vi "PH_BL-Master.ProcEvents.vi"(0 "i ref in":refnum<vi>, 5 "error in (no error)":errorcluster) -> (14 "i ref out":refnum<vi>, 19 "error out":errorcluster)   [LabVIEW 2014, in "PH_BL-Master.lvlib"]
doc: "This method is used to define the events the object will listen to. Add your own events here."
uses:
  PH_BL-Master.lvlib
  CSCore/BaseProcess/BaseProcess.event definition.ctl
  CSCore/CAEObj/CAEObj.event definition.ctl
  CSCore/BaseProcess/BaseProcess.descriptor string definition.ctl
  CSCore/BaseProcess/BaseProcess.lvlib
  CSCore/CAEObj/CAEObj.lvlib
  PH_Common/PH_Common.lvlib
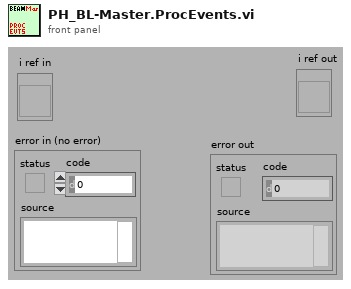
[diagram p1: front panel]
types:
  T1 = typedef "BaseProcess.lvlib/BaseProcess.event definition.ctl" = cluster{"CAEEvtDef":T2, "Data Descriptor":T3}
  T2 = typedef "CAEObj.lvlib/CAEObj.event definition.ctl" = cluster{"URL":string, "enable":bool, "ignoreResID":bool}
  T3 = typedef "BaseProcess.lvlib/BaseProcess.descriptor string definition.ctl" = string
  T4 = typedef "PH_BL-Master.lvlib/PH_BL-Master.i attribute.ctl" = cluster{"Remote controlled":bool, "Boolean Condition Service Subscriber":refnum<vi>[], "Picture Condition Service Subscriber":refnum<vi>[], "R2S":cluster{"GUI Ref":refnum<vi>, "State":bool}, "Vacua":cluster{"GUI Ref":refnum<vi>, "Limit":dbl, "Curr Value":dbl, "in range":bool}[], "O2 Inspection":cluster{"GUI Ref":refnum<vi>, "Concentration":dbl, "State":T5}[], "Boolean Status Service Subscriber":cluster{"GUI Ref":refnum<vi>, "Status":T5, "no Link?":bool, "Status Subscriber Class":T6}[], "Picture Status Service Subscriber":cluster{"GUI Ref":refnum<vi>, "Status":T5, "no Link?":bool, "Status Subscriber Class":T6}[], "6P 4Q Service Subscriber":cluster{"GUI Ref":refnum<vi>, "Selector":T7, "no Link?":bool}[], "Index of latest 6P 4Q changing Instance":i32, "Index of latest Picture Status changing Instance":i32, "Index of latest Boolean Status changing Instance":i32, "Vision ID on same Node":string, "Start Phase over?":bool, "GUI Ref Delete":refnum<vi>}
  T5 = typedef "PH_StatusHandler.lvlib/PH_StatusHandler.Status.ctl" = i16
  T6 = typedef "PH_BL-Master.lvlib/PH_BL-Master.Status Subscriber Class.ctl" = enum16{"unknown", "Switch", "BB", "6P Switch", "Switch GUI", "Switch and 6P State", "Force Sensor"}
  T7 = typedef "PH_4_Pos_Selector.lvlib/PH_4_Pos_Selector.Position Selector.ctl" = u16
  T8 = cluster{"GUI Ref":refnum<vi>, "Limit":dbl, "Curr Value":dbl, "in range":bool}[]
  T9 = cluster{"GUI Ref":refnum<vi>, "Selector":T7, "no Link?":bool}[]
  T10 = cluster{"GUI Ref":refnum<vi>, "Concentration":dbl, "State":T5}[]
  T11 = cluster{"GUI Ref":refnum<vi>, "Status":T5, "no Link?":bool, "Status Subscriber Class":T6}[]
  T12 = typedef "PH_Common.lvlib/PH_DIM.Event Declarer.ctl" = cluster{"Service Name":string, "Selector":string}
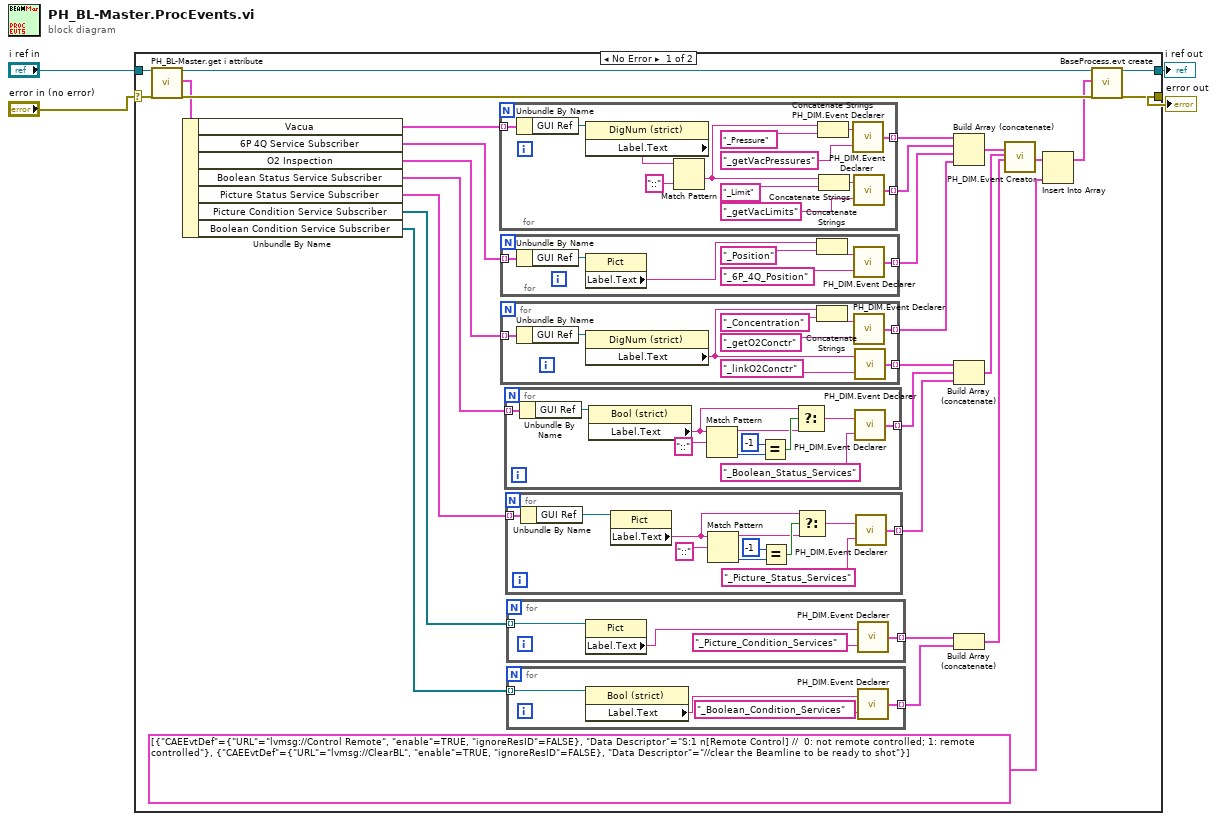
[diagram p0: block diagram]
diagram:
  n1 = case shown="No Error" "error in (no error)" {
    selector: "error in (no error)" -> [w23 w93]
    tunnel: [w33 w93] -> w4
    tunnel: [w32 w94] -> w3
    tunnel: "i ref in" -> [w31 w94]
    frame No Error {
      n2 = call "PH_BL-Master.get i attribute.vi"("i ref in"=w31, "error in (no error)"=w23) -> ("i ref out"=w30:refnum<vi>, "i attribute"=w28:T4, "error out"=w29:errorcluster)  [unwired: 15 in]
      n3 = Unbundle By Name(w28) -> ("Vacua"=w27:T8, "6P 4Q Service Subscriber"=w9:T9, "O2 Inspection"=w14:T10, "Boolean Status Service Subscriber"=w7:T11, "Picture Status Service Subscriber"=w5:T11, "Picture Condition Service Subscriber"=w15:refnum<vi>[], "Boolean Condition Service Subscriber"=w11:refnum<vi>[])
      n4 = for {
        tunnel: w27 -> [w92] mode=indexing
        tunnel: [w89] -> w18 mode=indexing
        tunnel: [w84] -> w17 mode=indexing
        n5 = Unbundle By Name(w92) -> ("GUI Ref"=w83:refnum<vi>)
        n6 = property class="DigNum (strict)"(reference=w83) -> ("Label.Text"=w82:string)  [unwired: 1 in, 2 out]
        n7 = Match Pattern(string=w82, regular expression="::") -> (after substring=w80:string)  [unwired: 1 in, 3 out]
        n8 = Concatenate Strings(w80, "_Pressure" ("string")) -> (w90:string)
        n9 = Concatenate Strings(w80, "_Limit" ("string")) -> (w86:string)
        n10 = call "PH_DIM.Event Declarer.vi"("Selector"="_getVacPressures", "Service Name"=w90) -> ("declared DIM Event"=w89:T12)
        n11 = call "PH_DIM.Event Declarer.vi"("Selector"="_getVacLimits", "Service Name"=w86) -> ("declared DIM Event"=w84:T12)
      }
      n12 = for {
        tunnel: [w49] -> w8 mode=indexing
        tunnel: w9 -> [w46] mode=indexing
        n13 = Unbundle By Name(w46) -> ("GUI Ref"=w48:refnum<vi>)
        n14 = property class="Pict"(reference=w48) -> ("Label.Text"=w47:string)  [unwired: 1 in, 2 out]
        n15 = Concatenate Strings(w47, "_Position" ("string")) -> (w51:string)
        n16 = call "PH_DIM.Event Declarer.vi"("Selector"="_6P_4Q_Position", "Service Name"=w51) -> ("declared DIM Event"=w49:T12)
      }
      n17 = for {
        tunnel: [w78] -> w21 mode=indexing
        tunnel: w14 -> [w73] mode=indexing
        tunnel: [w74] -> w16 mode=indexing
        n18 = Unbundle By Name(w73) -> ("GUI Ref"=w72:refnum<vi>)
        n19 = property class="DigNum (strict)"(reference=w72) -> ("Label.Text"=w71:string)  [unwired: 1 in, 2 out]
        n20 = Concatenate Strings(w71, "_Concentration" ("string")) -> (w77:string)
        n21 = call "PH_DIM.Event Declarer.vi"("Selector"="_getO2Conctr", "Service Name"=w77) -> ("declared DIM Event"=w74:T12)
        n22 = call "PH_DIM.Event Declarer.vi"("Selector"="_linkO2Conctr", "Service Name"=w71) -> ("declared DIM Event"=w78:T12)
      }
      n23 = for {
        tunnel: [w65] -> w10 mode=indexing
        tunnel: w7 -> [w63] mode=indexing
        n24 = Unbundle By Name(w63) -> ("GUI Ref"=w64:refnum<vi>)
        n25 = property class="Bool (strict)"(reference=w64) -> ("Label.Text"=w57:string)  [unwired: 1 in, 2 out]
        n26 = Match Pattern(string=w57, regular expression="::") -> (before substring=w60:string, offset past match=w59:i32)  [unwired: 1 in, 2 out]
        n27 = Equal?(x=-1 ("y"), y=w59) -> (x = y?=w61:bool)
        n28 = Select(t=w57, s=w61, f=w60) -> (s? t:f=w56:string)
        n29 = call "PH_DIM.Event Declarer.vi"("Selector"="_Boolean_Status_Services", "Service Name"=w56) -> ("declared DIM Event"=w65:T12)
      }
      n30 = for {
        tunnel: [w43] -> w6 mode=indexing
        tunnel: w5 -> [w41] mode=indexing
        n31 = Unbundle By Name(w41) -> ("GUI Ref"=w42:refnum<vi>)
        n32 = property class="Pict"(reference=w42) -> ("Label.Text"=w35:string)  [unwired: 1 in, 2 out]
        n33 = Match Pattern(string=w35, regular expression="::") -> (before substring=w38:string, offset past match=w37:i32)  [unwired: 1 in, 2 out]
        n34 = Equal?(x=-1 ("y"), y=w37) -> (x = y?=w39:bool)
        n35 = Select(t=w35, s=w39, f=w38) -> (s? t:f=w34:string)
        n36 = call "PH_DIM.Event Declarer.vi"("Selector"="_Picture_Status_Services", "Service Name"=w34) -> ("declared DIM Event"=w43:T12)
      }
      n37 = for {
        tunnel: w15 -> [w70] mode=indexing
        tunnel: [w67] -> w13 mode=indexing
        n38 = property class="Pict"(reference=w70) -> ("Label.Text"=w68:string)  [unwired: 1 in, 2 out]
        n39 = call "PH_DIM.Event Declarer.vi"("Selector"="_Picture_Condition_Services", "Service Name"=w68) -> ("declared DIM Event"=w67:T12)
      }
      n40 = for {
        tunnel: w11 -> [w55] mode=indexing
        tunnel: [w52] -> w12 mode=indexing
        n41 = property class="Bool (strict)"(reference=w55) -> ("Label.Text"=w53:string)  [unwired: 1 in, 2 out]
        n42 = call "PH_DIM.Event Declarer.vi"("Selector"="_Boolean_Condition_Services", "Service Name"=w53) -> ("declared DIM Event"=w52:T12)
      }
      n43 = Build Array (concatenate)(w18, w17, w8, w16) -> (w19:T12[])
      n44 = Build Array (concatenate)(w21, w10, w6) -> (w20:T12[])
      n45 = Build Array (concatenate)(w13, w12) -> (w22:T12[])
      n46 = call "PH_DIM.Event Creator.vi"("Trendmessage Services"=w19, "Status Services"=w20, "condition Services"=w22) -> ("DIM Service Events"=w26:T1[])  [unwired: 16 in]
      n47 = Insert Into Array(array=w26, new element=T1[] [{"CAEEvtDef"={"URL"="lvmsg://Control Remote", "enable"=TRUE, "ignoreResID"=FALSE}, "Data Descriptor"="S:1 n[Remote Control] //  0: not remote controlled; 1: remote controlled"}, {"CAEEvtDef"={"URL"="lvmsg://ClearBL", "enable"=TRUE, "ignoreResID"=FALSE}, "Data Descriptor"="//clear the Beamline to be ready to shot"}] ("new events")) -> (w24:T1[])  [unwired: 1 in]
      n48 = call "BaseProcess.evt create.vi"("i ref in"=w30, "newEvents"=w24, "error in (no error)"=w29) -> ("i ref out"=w32:refnum<vi>, "error out"=w33:errorcluster)  [unwired: 13 in, 2 out]
    }
    frame Error {
    }
  }
  "i ref out" <- w3
  "error out" <- w4
